vi "crit6.vi"(6 "Array":i16[](array[numeric])) -> ()   [LabVIEW 2010]
panel:
  out "output cluster":cluster{i32[], i16[]}
  out "порог":dbl
  out "XY Graph":cluster{i32[], i16[]}[](graph)
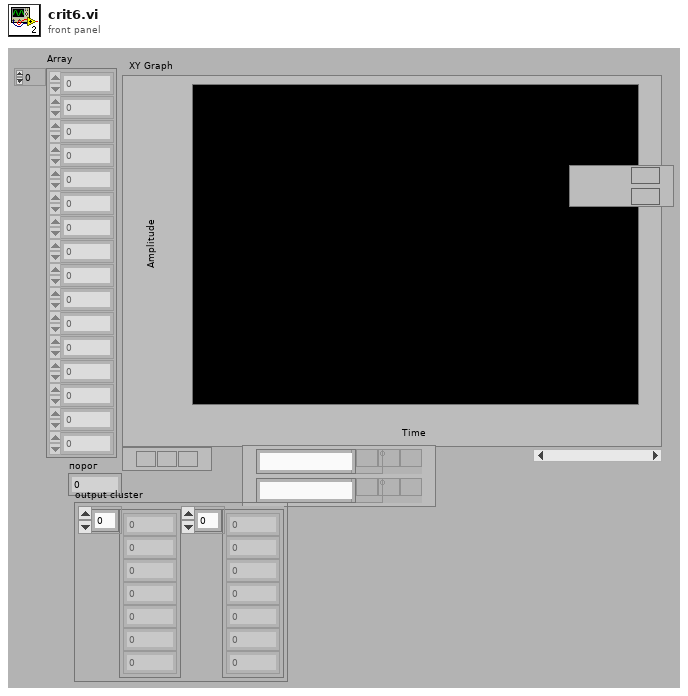
[diagram p1: front panel]
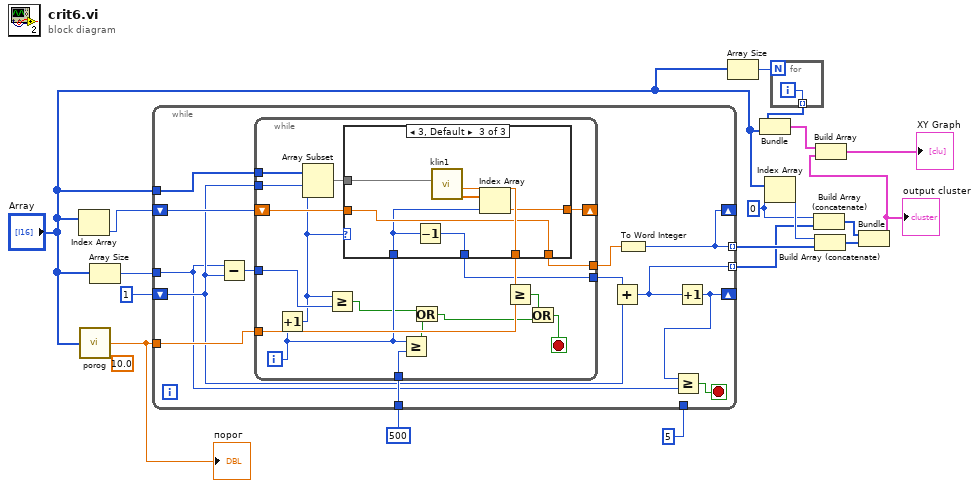
[diagram p0: block diagram]
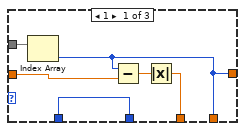
[diagram p2: hidden frame]
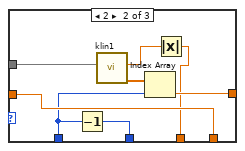
[diagram p3: hidden frame]
diagram:
  (unwired) 10.0 ("Numeric")
  w5 = 0 ("element")
  n1 = Index Array(array="Array") -> (element=w4:i16)  [unwired: 1 in]
  n2 = call "porog.vi"("Array"="Array") -> ("Numeric"=w1:dbl)
  "порог" <- w1
  n3 = Array Size(array="Array") -> (size(s)=w2:i32)
  n4 = while {
    tunnel: w1 -> [w31]
    tunnel: "Array" -> [w26]
    shift-right: [w20] -> _
    shift-left: 1 -> [w22]
    tunnel: 5 -> [_]
    tunnel: 500 -> [w28]
    tunnel: [w25] -> w9 mode=indexing
    tunnel: [w23] -> w7 mode=indexing
    shift-right: [w25] -> _
    shift-left: w4 -> [w24]
    tunnel: w2 -> [w19]
    stop <- w29 stop-if-true
    n5 = Subtract(x=w19, y=w22) -> (x-y=w21:i32)
    n6 = while {
      tunnel: w26 -> [w49]
      tunnel: w31 -> [w47]
      tunnel: [w37] -> w30
      tunnel: w28 -> [w46]
      shift-right: [w43] -> _
      shift-left: w24 -> [w40]
      tunnel: w22 -> [w42]
      tunnel: [w39] -> w27
      tunnel: w21 -> [w36]
      i -> [w38]
      stop <- w44 stop-if-true
      n7 = Increment(x=w38) -> (x+1=w35:i32)
      n8 = Array Subset(array=w49, index=w42, length=w35) -> (w41:i16[])
      n9 = Greater Or Equal?(x=w35, y=w36) -> (x >= y?=w34:bool)
      n10 = case shown="3, Default" w35 {
        tunnel: [w54 w56 w70] -> w48
        tunnel: [w51 w61 w68] -> w43
        tunnel: w41 -> [w55 w63 w67]
        tunnel: w40 -> [w52 w60 w66]
        tunnel: [w51 w60 w66] -> w39
        tunnel: w38 -> [w50 w59 w65]
        tunnel: [w50 w58 w64] -> w37
        frame 1 {
          n11 = Index Array(array=w55) -> (element=w51:i16)  [unwired: 1 in]
          n12 = Subtract(x=w51, y=w52) -> (x-y=w53:dbl)
          n13 = Absolute Value(x=w53) -> (abs(x)=w54:dbl)
        }
        frame 2 {
          n14 = Decrement(x=w59) -> (x-1=w58:i32)
          n15 = call "klin1.vi"("Array"=w63) -> ("line"=w62:dbl[], "наклон"=w57:dbl)  [unwired: 3 in, 2 out]
          n16 = Index Array(array=w62, index=w59) -> (element=w61:dbl)
          n17 = Absolute Value(x=w57) -> (abs(x)=w56:dbl)
        }
        frame 3, Default {
          n18 = Decrement(x=w65) -> (x-1=w64:i32)
          n19 = call "klin1.vi"("Array"=w67) -> ("line"=w69:dbl[], "max отклонение"=w70:dbl)  [unwired: 3 in, 2 out]
          n20 = Index Array(array=w69, index=w65) -> (element=w68:dbl)
        }
      }
      n21 = Greater Or Equal?(x=w38, y=w46) -> (x >= y?=w33:bool)
      n22 = Or(x=w34, y=w33) -> (x .or. y?=w32:bool)
      n23 = Greater Or Equal?(x=w48, y=w47) -> (x >= y?=w45:bool)
      n24 = Or(x=w45, y=w32) -> (x .or. y?=w44:bool)
    }
    n25 = Add(x=w30, y=w22) -> (x+y=w23:i32)
    n26 = To Word Integer(number=w27) -> (16bit integer=w25:i16)
    n27 = Increment(x=w23) -> (x+1=w20:i32)
    n28 = Greater Or Equal?(x=w20, y=w19) -> (x >= y?=w29:bool)
  }
  n29 = Array Size(array="Array") -> (size(s)=w11:i32)
  n30 = Index Array(array="Array", index=w5) -> (element=w10:i16)
  n31 = for {
    N: w11 -> [_]
    tunnel: [w71] -> w12 mode=indexing
    i -> [w71]
  }
  n32 = Bundle(w12, "Array"="Array") -> (w15:cluster{i32[], "Array":i16[]})  [unwired: 1 in]
  n33 = Build Array (concatenate)(w5, w7) -> (w6:i32[])
  n34 = Build Array (concatenate)(w10, w9) -> (w8:i16[])
  n35 = Bundle(w6, w8) -> (w14:cluster{i32[], i16[]})  [unwired: 1 in]
  "output cluster" <- w14
  n36 = Build Array(w15, w14) -> (→"XY Graph":cluster{i32[], "Array":i16[]}[])
